vi "Laboratory_practice4.vi"() -> ()   [LabVIEW 2022 SP3]
panel:
  out "Sine Graph":dbl[](graph)
  in  "Max degree":dbl
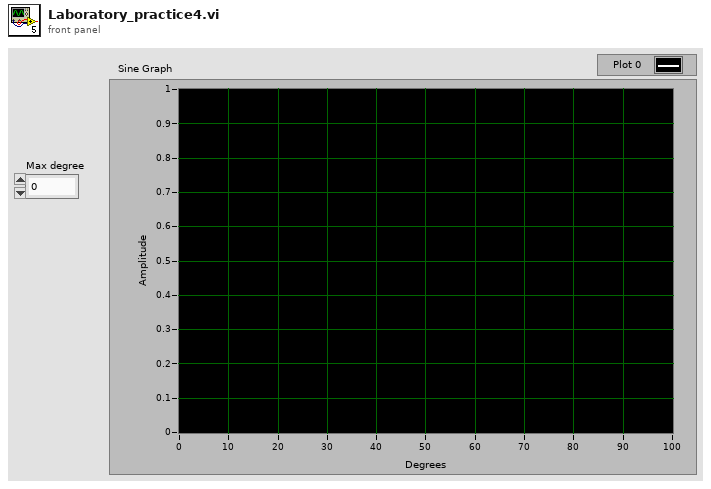
[diagram p1: front panel]
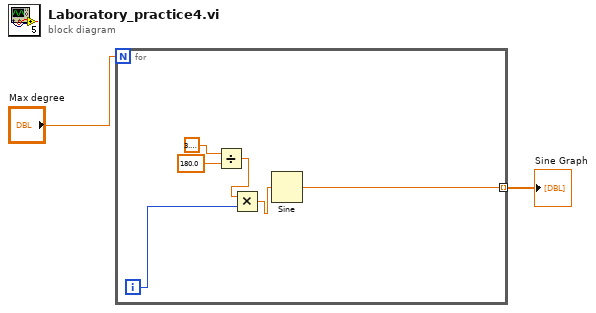
[diagram p0: block diagram]
diagram:
  n1 = for {
    N: "Max degree" -> [_]
    tunnel: [w8] -> w1 mode=indexing
    i -> [w7]
    n2 = Divide(x=3.141592653589793, y=180.0) -> (x/y=w3:dbl)
    n3 = Multiply(x=w3, y=w7) -> (x*y=w6:dbl)
    n4 = Sine(x=w6) -> (sin(x)=w8:dbl)
  }
  "Sine Graph" <- w1
